vi "test Parse System Definition to Create Tx Execution Units.vi"(8 "error in":errorcluster, 11 "TestCase in":refnum<class "Engine.lvclass">) -> (0 "error out":errorcluster, 3 "TestCase out":refnum<class "Engine.lvclass">)   [LabVIEW 2020, in "Engine.lvclass"]
uses:
  Engine.lvclass
  Engine/Implementation/Execution Unit Factory/Execution Unit Factory.lvclass
  Engine/Implementation/Tx Acyclic Labels Execution Unit/Tx Acyclic Labels Execution Unit.lvclass
  Engine/Implementation/Tx Scheduled Labels Execution Unit/Tx Scheduled Labels Execution Unit.lvclass
  Shared/RT Hardware Channel Settings.ctl
  Shared/RT Label Settings.ctl
  Shared/Label.ctl
  Shared/RT Parameters.ctl
  Shared/Parameter Definition.ctl
  <vilib>/NI/NI VeriStand Encoding and Decoding/Encoding.ctl
  <vilib>/NI VeriStand/Custom Device API/Custom Device Item Ref.ctl
  Shared/Transfer Type.ctl
  <vilib>/NI VeriStand/Custom Device API/Data Reference.ctl
  Engine/Implementation/Tx Scheduled Labels Execution Unit/Tx Scheduled Labels Execution Unit.lvclass/Tx Scheduled Labels Execution Unit.ctl
  Engine/Implementation/Tx Acyclic Labels Execution Unit/Tx Acyclic Labels Execution Unit.lvclass/Tx Acyclic Labels Execution Unit.ctl
  <vilib>/addons/_JKI Toolkits/VI Tester/TestCase.llb/TestCase.lvclass
  niveristand-custom-device-testing-tools/VeriStandTestUtilities/VeriStandTestUtilities.lvlib
  Scripting/AIM/AIM ARINC 429 Scripting.lvlib
  C:/Program Files (x86)/National Instruments/LabVIEW 2020/vi.lib/addons/_JKI Toolkits/VI Tester/TestCase.llb/TestCase.lvclass
  C:/dev/git/niveristand-aim-arinc429-custom-device/Source/Custom Device Support/Tests/Unit/Execution/Engine/Engine.lvclass
  <vilib>/NI VeriStand/Custom Device API/Custom Device API.lvlib
  <vilib>/NI/NI VeriStand Encoding and Decoding/Encoding and Decoding.lvlib
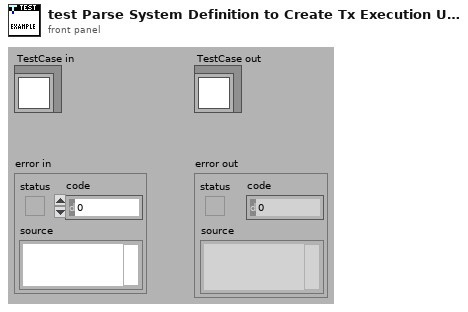
[diagram p1: front panel]
types:
  T1 = typedef "RT Hardware Channel Settings.ctl" = cluster{"channel #":u16, "channel handle":u64, "labels settings for RT":T2[]}
  T2 = typedef "RT Label Settings.ctl" = cluster{"Name":string, "xmlName":string, "label":T3, "transfer period":u32, "SDI_Enabled":bool, "SDI":u8, "parameter driver data":T4, "transfer type":T8, "has timestamp?":bool, "Label Disable/Trigger Channel Reference":T7, "Message Handle":u64, "Initialized?":bool, "Word Initial Raw Value":u32, "Label Timestamp Channel Data Reference":T9, "disabled":bool}
  T3 = typedef "Label.ctl" = u8
  T4 = typedef "RT Parameters.ctl" = cluster{"parameter definitions":T5[], "Tx parameter refs":T7[]}
  T5 = typedef "Parameter Definition.ctl" = cluster{"start index":i32, "size":i32, "encoding":T6, "signed":bool, "scale multiplier":dbl, "scale offset":dbl, "default value":dbl}
  T6 = typedef "Encoding and Decoding.lvlib/Encoding.ctl" = enum16{"BNR", "BCD", "Discrete"}
  T7 = typedef "Custom Device API.lvlib/Custom Device Item Ref.ctl" = u64
  T8 = typedef "Transfer Type.ctl" = enum16{"Scheduled", "Acyclic", "Block", "Strobe"}
  T9 = typedef "Custom Device API.lvlib/Data Reference.ctl" = i32
  T10 = typedef "AIM ARINC 429 Engine.lvlib/Interfaces.lvlib/Execution Unit Information.ctl" = cluster{"Execution Unit":refnum<class "Execution Unit.lvclass">, "Incoming Channels":T7[], "Outgoing Channels":T7[], "ReadWrite Channels":T7[]}
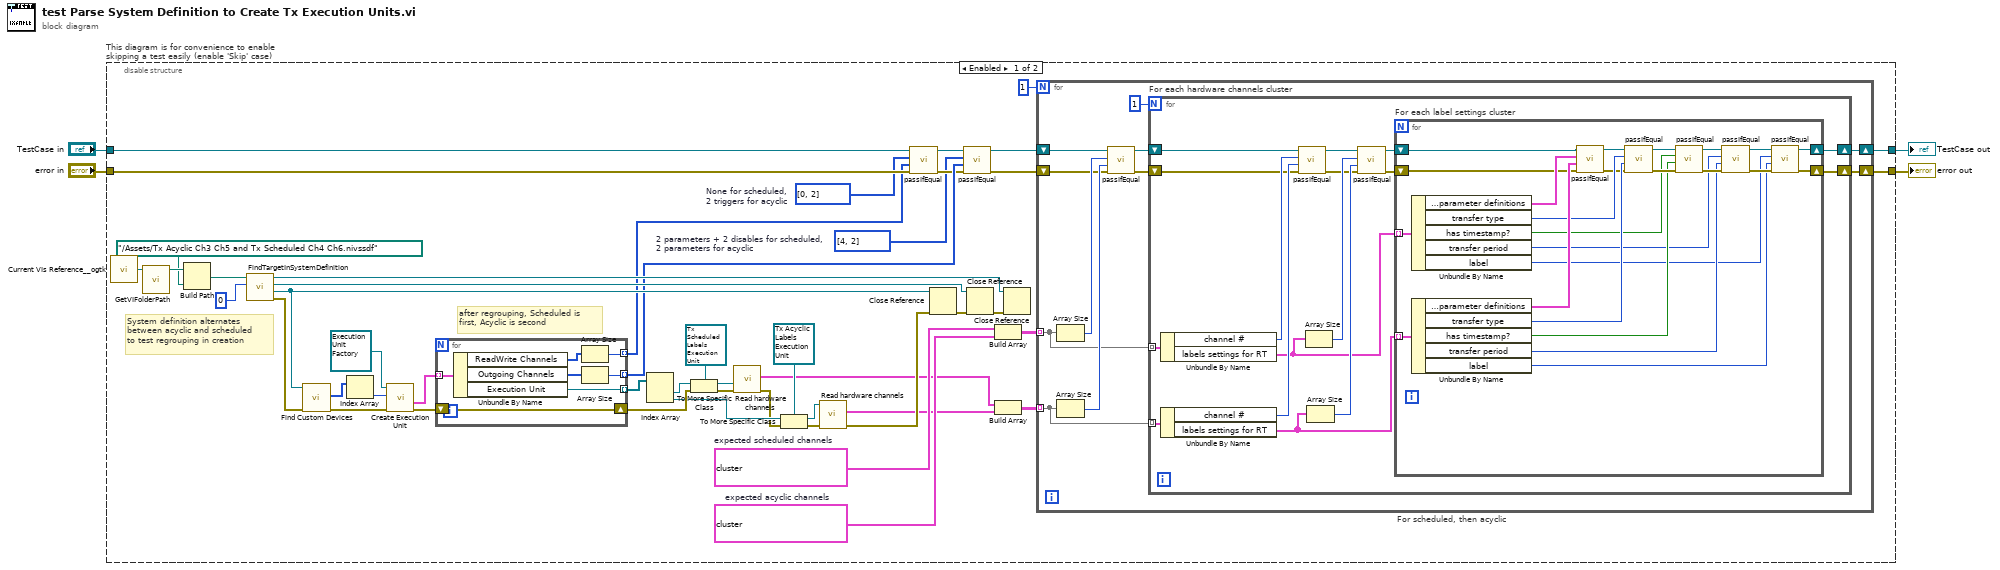
[diagram p0: block diagram]
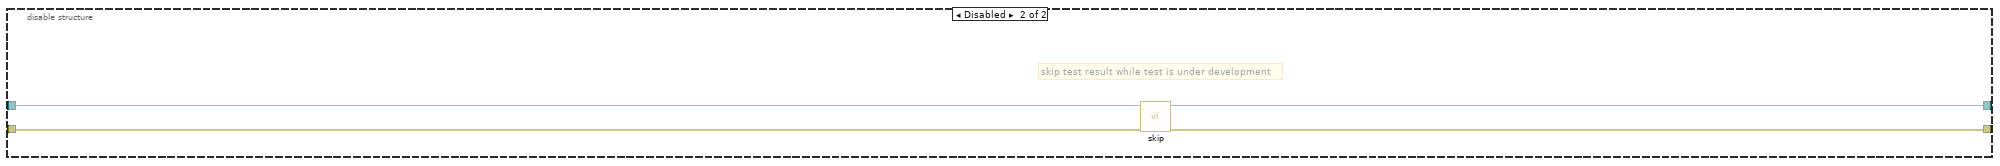
[diagram p2: hidden frame]
diagram:
  n1 = disable-structure "This diagram is for convenience to enable skipping a test easily (enable 'Skip' case)" shown="Enabled" {
    disable-tunnel: "TestCase in" -> [w52 w114]
    disable-tunnel: [w40 w112] -> w1
    disable-tunnel: [w39 w113] -> w3
    disable-tunnel: "error in" -> [w51 w111]
    frame Enabled {
      w9 = T1[] [{"channel #"=3, "channel handle"=0, "labels settings for RT"=[{"Name"="label 81", "xmlName"="", "label"=81, "transfer period"=10, "SDI_Enabled"=FALSE, "SDI"=0, "parameter driver data"={"parameter definitions"=[{"start index"=10, "size"=19, "encoding"=enum."BNR", "signed"=TRUE, "scale multiplier"=1.0, "scale offset"=0.0, "default value"=0.0}], "Tx parameter refs"=[35]}, "transfer type"=enum."Acyclic", "has timestamp?"=FALSE, "Label Disable/Trigger Channel Reference"=36, "Message Handle"=0, "Initialized?"=TRUE, "Word Initial Raw Value"=0, "Label Timestamp Channel Data Reference"=0, "disabled"=FALSE}]}, {"channel #"=5, "channel handle"=0, "labels settings for RT"=[{"Name"="label 83", "xmlName"="", "label"=83, "transfer period"=30, "SDI_Enabled"=FALSE, "SDI"=0, "parameter driver data"={"parameter definitions"=[{"start index"=10, "size"=19, "encoding"=enum."BNR", "signed"=FALSE, "scale multiplier"=1.0, "scale offset"=0.0, "default value"=0.0}], "Tx parameter refs"=[45]}, "transfer type"=enum."Acyclic", "has timestamp?"=FALSE, "Label Disable/Trigger Channel Reference"=46, "Message Handle"=0, "Initialized?"=TRUE, "Word Initial Raw Value"=0, "Label Timestamp Channel Data Reference"=0, "disabled"=FALSE}]}]  # expected acyclic channels
      w11 = T1[] [{"channel #"=4, "channel handle"=0, "labels settings for RT"=[{"Name"="label 82", "xmlName"="", "label"=82, "transfer period"=20, "SDI_Enabled"=FALSE, "SDI"=0, "parameter driver data"={"parameter definitions"=[{"start index"=10, "size"=19, "encoding"=enum."BNR", "signed"=TRUE, "scale multiplier"=1.0, "scale offset"=0.0, "default value"=0.0}], "Tx parameter refs"=[40]}, "transfer type"=enum."Scheduled", "has timestamp?"=FALSE, "Label Disable/Trigger Channel Reference"=41, "Message Handle"=0, "Initialized?"=TRUE, "Word Initial Raw Value"=0, "Label Timestamp Channel Data Reference"=0, "disabled"=FALSE}]}, {"channel #"=6, "channel handle"=0, "labels settings for RT"=[{"Name"="label 84", "xmlName"="", "label"=84, "transfer period"=40, "SDI_Enabled"=FALSE, "SDI"=0, "parameter driver data"={"parameter definitions"=[{"start index"=10, "size"=19, "encoding"=enum."BNR", "signed"=FALSE, "scale multiplier"=1.0, "scale offset"=0.0, "default value"=0.0}], "Tx parameter refs"=[50]}, "transfer type"=enum."Scheduled", "has timestamp?"=FALSE, "Label Disable/Trigger Channel Reference"=51, "Message Handle"=0, "Initialized?"=TRUE, "Word Initial Raw Value"=0, "Label Timestamp Channel Data Reference"=0, "disabled"=FALSE}]}]  # expected scheduled channels
      w13 = i32[] [4, 2]  # 2 parameters + 2 disables for scheduled, 2 parameters for acyclic
      w14 = i32[] [0, 2]  # None for scheduled, 2 triggers for acyclic
      # "System definition alternates\nbetween acyclic and scheduled\nto test regrouping in creation"
      # "after regrouping, Scheduled is \nfirst, Acyclic is second"
      n2 = call <userlib>:"Current VIs Reference__ogtk.vi"() -> ("Current VI's reference"=w42:refnum<vi>)  [unwired: 5 in]
      n3 = call "GetVIFolderPath.vi"("VI Reference in"=w42) -> ("VI Folder Path out"=w43:path)  [unwired: 9 in, 1 out]
      n4 = Build Path(base path=w43, name or relative path=path "../Assets/Tx Acyclic Ch3 Ch5 and Tx Scheduled Ch4 Ch6.nivssdf" ("system definition path")) -> (appended path=w41:path)
      n5 = call "FindTargetInSystemDefinition.vi"("target index"=0 ("index"), "system definition path"=w41) -> ("error out"=w44:errorcluster, "Target"=w47:refnum<k24>, "Root"=w46:refnum<k24>, "System Definition"=w45:refnum<k24>)  [unwired: 6 in]
      n6 = call "Find Custom Devices.vi"("error in"=w44, "target in"=w47) -> ("error out"=w35:errorcluster, "AIM ARINC 429 custom devices"=w37:u64[])  [unwired: 7 in, 1 out]
      n7 = Index Array(array=w37) -> (element=w36:u64)  [unwired: 1 in]
      n8 = call-dynamic "Create Execution Unit.vi"("error in"=w35, "Item Ref"=w36, "Execution Unit Factory Implementation in"=refnum<class "Execution Unit Factory.lvclass"> refnum ("Communication Bus Template Interfaces:Implementation.lvlib:Execution Unit Factory.lvclass")) -> ("error out"=w32:errorcluster, "Asynchronous Execution Units"=w33:T10[])  [unwired: 5 in, 2 out]
      n9 = for {
        tunnel: w33 -> [w110] mode=indexing
        shift-right: [w109] -> w25
        shift-left: w32 -> [w109]
        tunnel: [w108] -> w26 mode=indexing
        tunnel: [w106] -> w31 mode=indexing
        tunnel: [w107] -> w12 mode=indexing
        n10 = Unbundle By Name(w110) -> ("ReadWrite Channels"=w104:T7[], "Outgoing Channels"=w105:T7[], "Execution Unit"=w108:refnum<class "Execution Unit.lvclass">)
        n11 = Array Size(array=w104) -> (size(s)=w107:i32)
        n12 = Array Size(array=w105) -> (size(s)=w106:i32)
      }
      n13 = Index Array(array=w26) -> (element #1=w23:refnum<class "Execution Unit.lvclass">, element #2=w22:refnum<class "Execution Unit.lvclass">)  [unwired: 2 in]
      n14 = To More Specific Class(target class=refnum<class "Tx Scheduled Labels Execution Unit.lvclass"> refnum ("Communication Bus Template Interfaces:Implementation.lvlib:Tx Scheduled Labels Execution Unit.lvclass"), reference=w23, error in=w25) -> (specific class reference=w20:refnum<class "Tx Scheduled Labels Execution Unit.lvclass">, error out=w19:errorcluster)
      n15 = call "Read hardware channels.vi"("error in (no error)"=w19, "Tx Scheduled Labels Execution Unit in"=w20) -> ("error out"=w18:errorcluster, "hardware channels"=w7:T1[])  [unwired: 7 in, 1 out]
      n16 = To More Specific Class(target class=refnum<class "Tx Acyclic Labels Execution Unit.lvclass"> refnum ("Communication Bus Template Interfaces:Implementation.lvlib:Tx Acyclic Labels Execution Unit.lvclass"), reference=w22, error in=w18) -> (specific class reference=w16:refnum<class "Tx Acyclic Labels Execution Unit.lvclass">, error out=w17:errorcluster)
      n17 = call "Read hardware channels.vi"("error in (no error)"=w17, "Tx Acyclic Labels Execution Unit in"=w16) -> ("error out"=w15:errorcluster, "hardware channels"=w6:T1[])  [unwired: 7 in, 1 out]
      n18 = call-dynamic "passIfEqual.vi"("error in (no error)"=w51, "y"=w12, "x"=w14, "TestCase in"=w52) -> ("error out"=w30:errorcluster, "TestCase out"=w28:refnum<class "Engine.lvclass">)  [unwired: 6 in]
      n19 = Close Reference(reference=w47, error in (no error)=w15) -> (error out=w49:errorcluster)
      n20 = call-dynamic "passIfEqual.vi"("error in (no error)"=w30, "y"=w31, "x"=w13, "TestCase in"=w28) -> ("error out"=w29:errorcluster, "TestCase out"=w27:refnum<class "Engine.lvclass">)  [unwired: 6 in]
      n21 = Close Reference(reference=w46, error in (no error)=w49) -> (error out=w48:errorcluster)
      n22 = Build Array(w11, w9) -> (w10:T1[][])
      n23 = Build Array(w7, w6) -> (w8:T1[][])
      n24 = Close Reference(reference=w45, error in (no error)=w48) -> ()  [unwired: 1 out]
      n25 = for "For scheduled, then acyclic" {
        N: 1 -> [_]
        tunnel: w8 -> [w55] mode=indexing
        tunnel: w10 -> [w54] mode=indexing
        shift-right: [w60] -> w39
        shift-left: w29 -> [w59]
        shift-right: [w61] -> w40
        shift-left: w27 -> [w58]
        n26 = Array Size(array=w54) -> (size(s)=w63:i32)
        n27 = Array Size(array=w55) -> (size(s)=w62:i32)
        n28 = call-dynamic "passIfEqual.vi"("error in (no error)"=w59, "y"=w62, "x"=w63, "TestCase in"=w58) -> ("error out"=w56:errorcluster, "TestCase out"=w57:refnum<class "Engine.lvclass">)  [unwired: 6 in]
        n29 = for "For each hardware channels cluster" {
          N: 1 -> [_]
          tunnel: w54 -> [w79] mode=indexing
          shift-right: [w65] -> w61
          shift-left: w57 -> [w76]
          shift-right: [w64] -> w60
          shift-left: w56 -> [w75]
          tunnel: w55 -> [w70] mode=indexing
          n30 = Unbundle By Name(w79) -> ("channel #"=w78:u16, "labels settings for RT"=w66:T2[])
          n31 = Unbundle By Name(w70) -> ("channel #"=w77:u16, "labels settings for RT"=w67:T2[])
          n32 = call-dynamic "passIfEqual.vi"("error in (no error)"=w75, "y"=w77, "x"=w78, "TestCase in"=w76) -> ("error out"=w71:errorcluster, "TestCase out"=w72:refnum<class "Engine.lvclass">)  [unwired: 6 in]
          n33 = Array Size(array=w66) -> (size(s)=w74:i32)
          n34 = Array Size(array=w67) -> (size(s)=w73:i32)
          n35 = call-dynamic "passIfEqual.vi"("error in (no error)"=w71, "y"=w73, "x"=w74, "TestCase in"=w72) -> ("error out"=w69:errorcluster, "TestCase out"=w68:refnum<class "Engine.lvclass">)  [unwired: 6 in]
          n36 = for "For each label settings cluster" {
            tunnel: w66 -> [w103] mode=indexing
            tunnel: w67 -> [w94] mode=indexing
            shift-right: [w83] -> w65
            shift-left: w68 -> [w96]
            shift-right: [w82] -> w64
            shift-left: w69 -> [w95]
            n37 = Unbundle By Name(w103) -> ("parameter driver data.parameter definitions"=w102:T5[], "transfer type"=w100:T8, "has timestamp?"=w89:bool, "transfer period"=w87:u32, "label"=w80:T3)
            n38 = Unbundle By Name(w94) -> ("parameter driver data.parameter definitions"=w101:T5[], "transfer type"=w99:T8, "has timestamp?"=w88:bool, "transfer period"=w86:u32, "label"=w81:T3)
            n39 = call-dynamic "passIfEqual.vi"("error in (no error)"=w95, "y"=w101, "x"=w102, "TestCase in"=w96) -> ("error out"=w97:errorcluster, "TestCase out"=w98:refnum<class "Engine.lvclass">)  [unwired: 6 in]
            n40 = call-dynamic "passIfEqual.vi"("error in (no error)"=w97, "y"=w99, "x"=w100, "TestCase in"=w98) -> ("error out"=w93:errorcluster, "TestCase out"=w92:refnum<class "Engine.lvclass">)  [unwired: 6 in]
            n41 = call-dynamic "passIfEqual.vi"("error in (no error)"=w93, "y"=w88, "x"=w89, "TestCase in"=w92) -> ("error out"=w91:errorcluster, "TestCase out"=w90:refnum<class "Engine.lvclass">)  [unwired: 6 in]
            n42 = call-dynamic "passIfEqual.vi"("error in (no error)"=w91, "y"=w86, "x"=w87, "TestCase in"=w90) -> ("error out"=w85:errorcluster, "TestCase out"=w84:refnum<class "Engine.lvclass">)  [unwired: 6 in]
            n43 = call-dynamic "passIfEqual.vi"("error in (no error)"=w85, "y"=w81, "x"=w80, "TestCase in"=w84) -> ("error out"=w82:errorcluster, "TestCase out"=w83:refnum<class "Engine.lvclass">)  [unwired: 6 in]
          }
        }
      }
    }
    frame Disabled {
      # "skip test result while test is under development"
      n44 = call <vilib>:"skip.vi"("error in (no error)"=w111, "TestCase in"=w114) -> ("error out"=w113:errorcluster, "TestCase out"=w112:refnum<class "Engine.lvclass">)  [unwired: 8 in]
    }
  }
  "error out" <- w3
  "TestCase out" <- w1
